vi "Write Buses.vi"(8 "error in (no error)":errorcluster, 10 "Buses":refnum<class "Bus_Access.lvclass">[](array[class]), 11 "Fault-Injection Bus in":refnum<class "Fault-Injection Bus.lvclass">) -> (0 "error out":errorcluster, 3 "Fault-Injection Bus out":refnum<class "Fault-Injection Bus.lvclass">)   [LabVIEW 2021, in "Fault-Injection Bus.lvclass"]
uses:
  Fault-Injection Bus.lvclass
  Fault-Injection Bus.lvclass/Fault-Injection Bus.ctl
  Omni-Bus/Bus Access/Bus_Access.lvclass
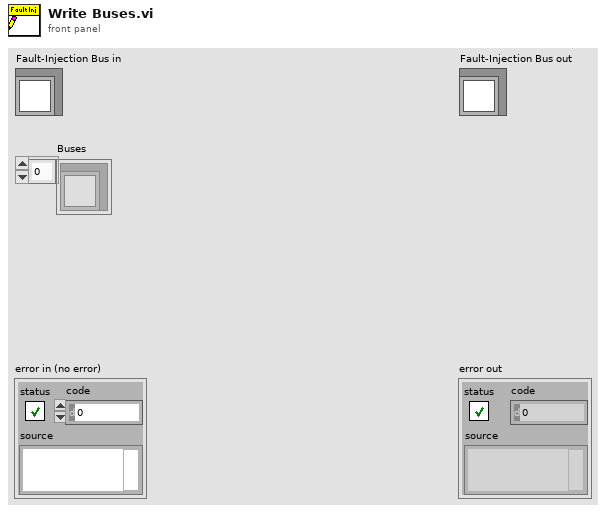
[diagram p1: front panel]
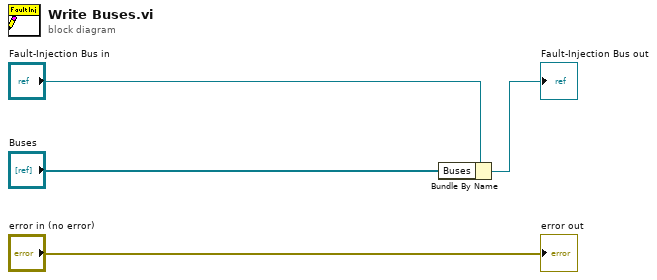
[diagram p0: block diagram]
diagram:
  n1 = Bundle By Name(cluster="Fault-Injection Bus in", "Buses"="Buses") -> (→"Fault-Injection Bus out":refnum<class "Fault-Injection Bus.lvclass">)
  "error out" <- "error in (no error)"
